vi "WPI_RobotDriveMotors_3005.vi"(8 "error in":errorcluster, 9 "RightSpeed":dbl, 10 "LeftSpeed":dbl, 11 "RobotDriveDevRef":T1={"DevStatus"={"status"=FALSE, "code"=0, "source"=""}, "Motors[]"=[], "Square Inputs"=FALSE, "Max Output"=1.0}) -> (0 "error out":errorcluster, 3 "RobotDriveDevRef":T1={"DevStatus"={"status"=FALSE, "code"=0, "source"=""}, "Motors[]"=[], "Square Inputs"=FALSE, "Max Output"=1.0})   [LabVIEW 2016, in "Drive System.lvlib"]
doc: "Determines the motor configuration and sends the speed values to the appropriate motors.\n\nThis software is licensed. Open the labview\\readme\\WPI Robotics Library Open Source License.txt file for more information."
uses:
  SubSystems/Drive/Drive System.lvlib
  <vilib>/Rock Robotics/WPI/RobotDrive/WPI_RobotDriveDevRef.ctl
  <vilib>/Rock Robotics/WPI/MotorControl/WPI_MotorControlDeviceRef.ctl
  <vilib>/Rock Robotics/WPI/MotorControl/WPI_MotorControlType.ctl
  <vilib>/Rock Robotics/SystemInterfaces/DIO/FPGA_DIOPWMChannel.ctl
  <vilib>/Rock Robotics/WPI/PWM/WPI_PWMDeadband.ctl
  SubSystems/Drive/Private/Raw Data.vi
  <vilib>/Rock Robotics/WPI/RobotDrive/WPI_RobotDriveSafetyCheck.vi
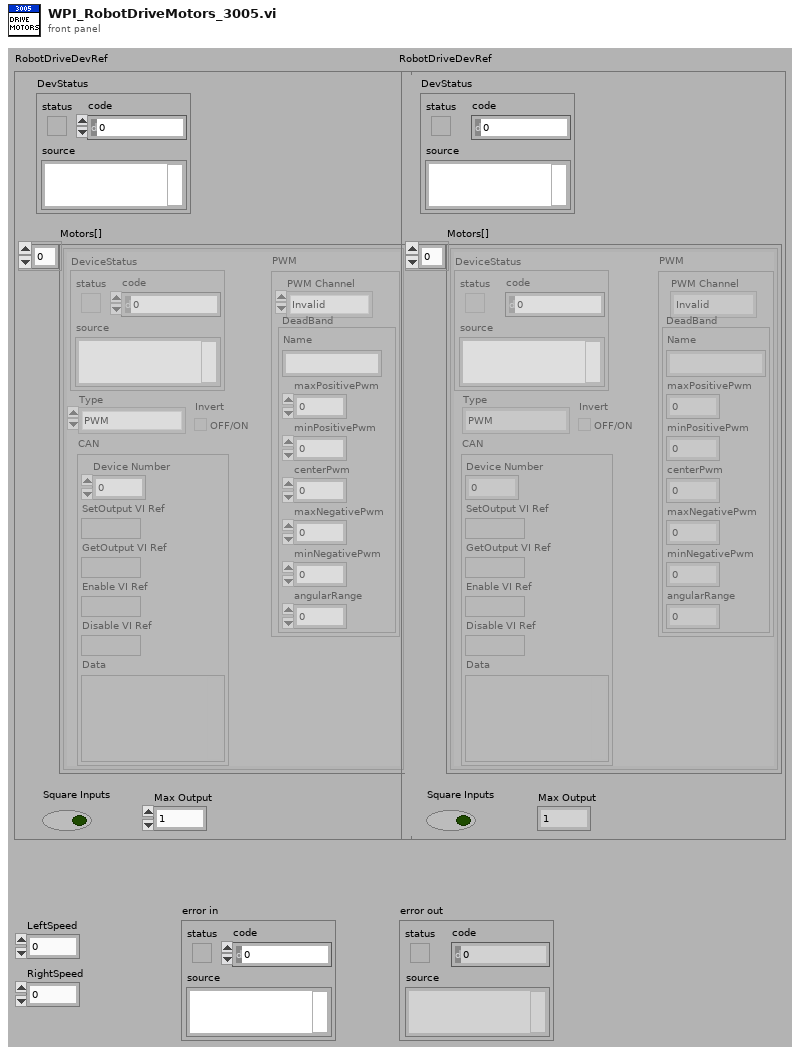
[diagram p1: front panel]
types:
  T1 = typedef "WPI_RobotDriveDevRef.ctl" = cluster{"DevStatus":errorcluster, "Motors[]":T2[], "Square Inputs":bool, "Max Output":dbl}
  T2 = typedef "WPI_MotorControlDeviceRef.ctl" = cluster{"DeviceStatus":errorcluster, "Type":T3, "PWM":cluster{"PWM Channel":T4, "DeadBand":T5}, "CAN":cluster{"Device Number":u8, "SetOutput VI Ref":variant, "GetOutput VI Ref":variant, "Enable VI Ref":variant, "Disable VI Ref":variant, "Data":variant}, "Invert":bool}
  T3 = typedef "WPI_MotorControlType.ctl" = enum16{"PWM", "CAN"}
  T4 = typedef "FPGA_DIOPWMChannel.ctl" = enum8{"PWM 0", "PWM 1", "PWM 2", "PWM 3", "PWM 4", "PWM 5", "PWM 6", "PWM 7", "PWM 8", "PWM 9", "PWM MXP 0", "PWM MXP 1", "PWM MXP 2", "PWM MXP 3", "PWM MXP 4", "PWM MXP 5", "PWM MXP 6", "PWM MXP 7", "PWM MXP 8", "PWM MXP 9", "Invalid"}
  T5 = typedef "WPI_PWMDeadband.ctl" = cluster{"Name":string, "maxPositivePwm":i32, "minPositivePwm":i32, "centerPwm":i32, "maxNegativePwm":i32, "minNegativePwm":i32, "angularRange":u16}
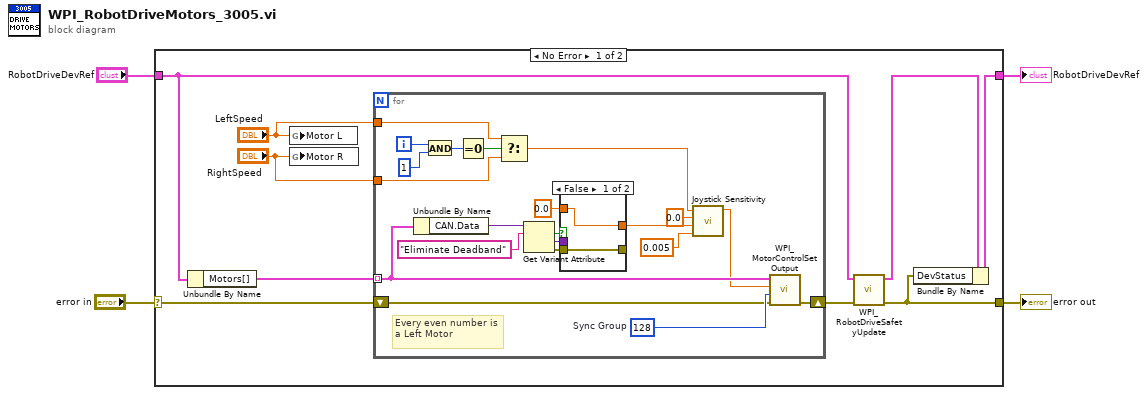
[diagram p0: block diagram]
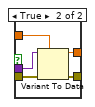
[diagram p2: hidden frame]
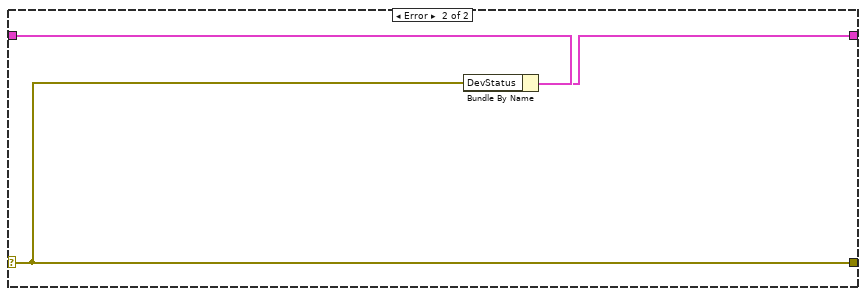
[diagram p3: hidden frame]
diagram:
  n1 = case shown="No Error" "error in" {
    selector: "error in" -> [w7 w42]
    tunnel: "RobotDriveDevRef" -> [w11 w44]
    tunnel: [w9 w43] -> w3
    tunnel: [w8 w42] -> w2
    frame No Error {
      n2 = Unbundle By Name(w11) -> ("Motors[]"=w13:T2[])
      n3 = global write "Raw Data.vi" "Motor L"("LeftSpeed") -> ()
      n4 = global write "Raw Data.vi" "Motor R"("RightSpeed") -> ()
      n5 = for {
        tunnel: w13 -> [w25] mode=indexing
        shift-right: [w29] -> w12
        shift-left: w7 -> [w28]
        tunnel: "LeftSpeed" -> [w27]
        tunnel: "RightSpeed" -> [w26]
        i -> [w34]
        w30 = u8 128  # Sync Group
        # "Every even number is a Left Motor"
        n6 = Unbundle By Name(w25) -> ("CAN.Data"=w24:variant)
        n7 = And(x=w34, y=1) -> (x .and. y?=w32:i32)
        n8 = Equal To 0?(x=w32) -> (x = 0?=w31:bool)
        n9 = Select(t=w27, s=w31, f=w26) -> (s? t:f=w16:dbl)
        n10 = Get Variant Attribute(Variant=w24, name="Eliminate Deadband") -> (found=w21:bool, value=w20:variant, error out=w22:errorcluster)  [unwired: 2 in, 1 out]
        n11 = case shown="False" w21 {
          tunnel: w22 -> [w35 w41]
          tunnel: [w36 w40] -> w17
          tunnel: w20 -> [_ w39]
          tunnel: 0.0 -> [w36 w38]
          tunnel: [w35 w37] -> _
          frame False {
          }
          frame True {
            n12 = Variant To Data(error in=w41, type=w38, Variant=w39) -> (data=w40:dbl, error out=w37:errorcluster)
          }
        }
        n13 = call "Joystick Sensitivity.vi"("joystick deadband"=0.005, "motor deadband (0.15)"=w17, "sensitivity (0.5)"=0.0, "x"=w16) -> ("y"=w14:dbl)  [unwired: 6 in, 1 out]
        n14 = call <vilib>:"WPI_MotorControlSetOutput.vi"("error in (no error)"=w28, "options"=w30, "Output"=w14, "MotorControlDevRef"=w25) -> ("error out"=w29:errorcluster)  [unwired: 7 out]
      }
      n15 = call <vilib>:"WPI_RobotDriveSafetyUpdate.vi"("error in (no error)"=w12, "RobotDriveDevRef"=w11) -> ("error out"=w8:errorcluster, "RobotDriveDevRef"=w10:T1)  [unwired: 8 out]
      n16 = Bundle By Name(cluster=w10, "DevStatus"=w8) -> (w9:T1)
    }
    frame Error {
      n17 = Bundle By Name(cluster=w44, "DevStatus"=w42) -> (w43:T1)
    }
  }
  "RobotDriveDevRef" <- w3
  "error out" <- w2
